vi "templates copy template.vi"(6 "username":string, 7 "POST Parameters":T1, 8 "error in":errorcluster, 9 "Keys in":T1, 10 "template":string, 11 "Connection Refnum":T2) -> (0 "error out":errorcluster, 1 "Parameters":T1, 3 "Connection Refnum":T2)   [LabVIEW 2011]
uses:
  SI.LIB/ODBC/SQL Controls/Connection Refnum.ctl
  Addons/internet/utils/keyedarr.llb/Keyed Array.ctl
  Addons/internet/utils/strutil.llb/Case Matching.ctl
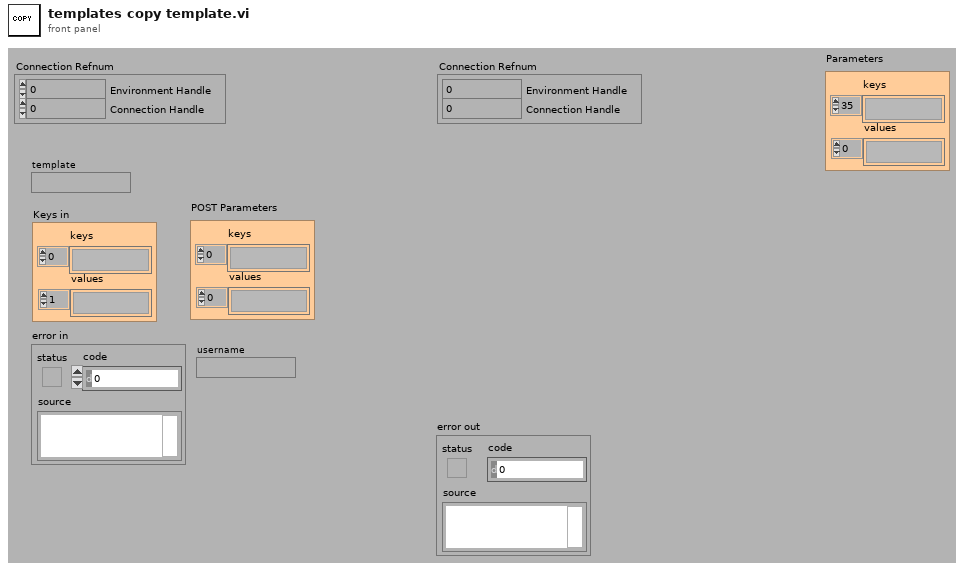
[diagram p1: front panel]
types:
  T1 = typedef "Keyed Array.ctl" = cluster{"keys":string[], "values":string[]}
  T2 = typedef "Connection Refnum.ctl" = cluster{"Environment Handle":i32, "Connection Handle":i32}
  T3 = typedef "Case Matching.ctl" = enum16{"a != A", "a == A", "system"}
  T4 = typedef "Template Record.ctl" = cluster{"ixTemplate":i32, "sxTemplateId":string, "sDescription":string, "sCreator":string, "tCreationDate":timestamp, "sModifier":string, "tModifiedDate":timestamp, "sType":string, "sStyle":string, "sFormat":string, "dWidth":dbl, "dHeight":dbl, "sFilename":string, "sScript":string, "sLayout":string, "sEditor":string, "sStyleProcess":string}
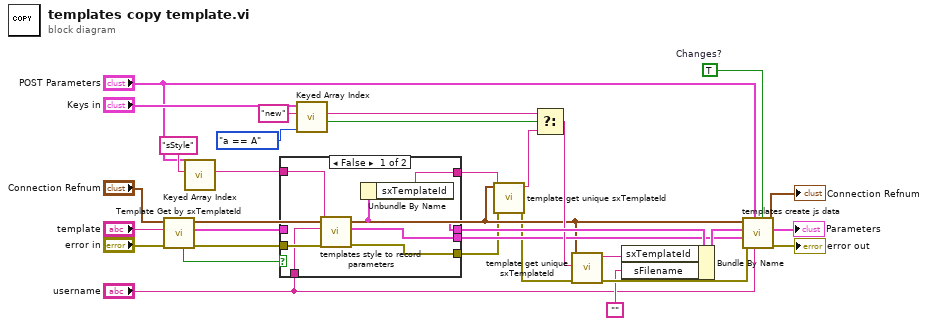
[diagram p0: block diagram]
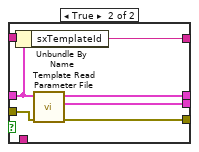
[diagram p2: hidden frame]
diagram:
  w10 = TRUE  # Changes?
  n1 = call "Template Get by sxTemplateId.vi"("error in (no error)"="error in", "sxTemplateId (\"\")"="template", "Connection Refnum"="Connection Refnum") -> ("error out"=w6:errorcluster, "Template Record"=w24:T4, "Connection Refnum"=w14:T2, "Data Present"=w7:bool)  [unwired: 5 out]
  n2 = call "Keyed Array Index.vi"("key"="sStyle", "array in"="POST Parameters") -> ("value"=w2:string)  [unwired: 2 in, 3 out]
  n3 = case shown="False" w7 {
    tunnel: [w33 w44] -> w31
    tunnel: w24 -> [_ w43]
    tunnel: [w32 w42] -> w19
    tunnel: [w35 w41] -> w15
    tunnel: w6 -> [w38 w40]
    tunnel: [w34 w39] -> w5
    tunnel: w2 -> [w37 _]
    tunnel: "username" -> [w36 _]
    frame False {
      n4 = call "templates style to record parameters.vi"("error in (no error)"=w38, "user"=w36, "template style"=w37) -> ("error out"=w34:errorcluster, "Parameters"=w35:T1, "Template Record"=w33:T4)  [unwired: 6 out]
      n5 = Unbundle By Name(w33) -> ("sxTemplateId"=w32:string)
    }
    frame True {
      n6 = Unbundle By Name(w43) -> ("sxTemplateId"=w42:string)
      n7 = call "Template Read Parameter File.vi"("error in (no error)"=w40, "Template Record"=w43) -> ("error out"=w39:errorcluster, "Parameters"=w41:T1, "updated Template Record"=w44:T4)  [unwired: 1 in, 6 out]
    }
  }
  n8 = call "Keyed Array Index.vi"("case matching (sensitive)"=Case_Matching."a == A", "key"="new", "array in"="Keys in") -> ("valid key"=w23:bool, "value"=w22:string)  [unwired: 1 in, 2 out]
  n9 = call "template get unique sxTemplateId.vi"("error in"=w5, "sxTemplateId proposed"=w19, "Connection Refnum"=w14) -> ("error out"=w4:errorcluster, "sxTemplateId"=w18:string)  [unwired: 7 out]
  n10 = Select(t=w22, s=w23, f=w18) -> (s? t:f=w20:string)
  n11 = call "template get unique sxTemplateId.vi"("error in"=w4, "sxTemplateId proposed"=w20, "Connection Refnum"=w14) -> ("error out"=w11:errorcluster, "sxTemplateId"=w21:string)  [unwired: 7 out]
  n12 = Bundle By Name(cluster=w31, "sxTemplateId"=w21, "sFilename"="") -> (w16:T4)
  n13 = call "templates create js data.vi"("Changes?"=w10, "sxUsername"="username", "POST Parameters"="POST Parameters", "error in (no error)"=w11, "template Parameters"=w15, "Template Record"=w16, "Connection Refnum"=w14) -> ("error out"=→"error out":errorcluster, "HTM Keys"=→"Parameters":T1, "Connection Refnum"=→"Connection Refnum":T2)  [unwired: 2 out]
